vi "host_chunk.vi"() -> ()   [LabVIEW 2020]
doc: "This example demonstrates how to continuously acquire buffered voltage measurements using a DAQmx device.\n\nFor instructions on how to connect your signals to the DAQ device, refer to your device documentation."
uses:
  <vilib>/DAQmx/read.llb/DAQmx Read (Analog Wfm 1Chan NSamp).vi
  <vilib>/DAQmx/create/channels.llb/DAQmx Create Channel (AI-Voltage-Basic).vi
  <vilib>/DAQmx/configure/timing.llb/DAQmx Timing (Sample Clock).vi
  <vilib>/FPGAPlugInAG/cRIO-9040/niLvFpga_Open_cRIO-9040.vi
  <vilib>/rvi/interface/common/dynamic/niFpgaDynamicAddResources.vi
  <vilib>/Utility/error.llb/Error Cluster From Error Code.vi
  <vilib>/rvi/errors/niLvFpgaAdjustHostInterfaceError.vi
  <vilib>/FPGAPlugInAG/Dynamic/niLvFpga_Run_Dynamic.vi
  <vilib>/RVI Host/nirviSupport.llb/nirviErrorClusterFromErrorCode.vi
  <vilib>/DAQmx/miscellaneous.llb/DAQmx Fill In Error Info.vi
  <vilib>/FPGAPlugInAG/Dynamic/niLvFpga_Close_Dynamic.vi
  <vilib>/rvi/interface/nirviOpenFPGA/nirviOpenFPGA.xnode
  FPGA Bitfiles/testDMA_9040_chunk_v1001.lvbitx
  <vilib>/rvi/interface/nirviReadWriteControl/nirviReadWriteControl.xnode
  <vilib>/rvi/interface/nirviMethod/nirviMethod.xnode
  <vilib>/rvi/interface/nirviCloseFPGA/nirviCloseFPGA.xnode
  <resource>/objmgr/daqmx.rc
  <vilib>/rvi/interface/Simulation/niFpgaSimulationCallBeginRW.vi
  <vilib>/rvi/errors/niLvFpgaMergeErrorWithErrorCode.vi
  NiFpgaLv.dll
  <vilib>/FPGAPlugInAG/Dynamic/niLvFpga_WriteFifo_Dynamic.vi
  <vilib>/FPGAPlugInAG/Dynamic/niLvFpga_ReadFifo_Dynamic.vi
  <vilib>/rvi/interface/nirviMethod/StockFPGA_InlinedMethodWaitForSingleIRQ.vi
  <vilib>/FPGAPlugInAG/Dynamic/niLvFpga_WaitOnIrq_Dynamic.vi
  <vilib>/FPGAPlugInAG/Dynamic/niLvFpga_AcknowledgeIrq_Dynamic.vi
panel:
  out "dma read time uS":u32
  out "AvailSampPerChan":u32
  out "write DMA timeout count":i16
  out "uS elapsed":cluster{u32, u32}(graph)
  out "Timed Out":bool
  out "error out":errorcluster
  in  "Stop":bool
  out "Waveform Graph":dbl[][](graph)
  in  "Number of Samples":i32=100
  in  "Sample Rate":dbl=1000.0
  in  "Sample Clock Source":tag="OnboardClock"
  in  "Terminal Configuration":i32(ring)=-1 items=["default"=-1, "RSE"=10083, "NRSE"=10078, "Differential"=10106, "Pseudodifferential"=12529]
  in  "Max Voltage":dbl=5.0
  in  "Min Voltage":dbl=-5.0
  in  "Physical Channel":tag="Mod1/ai0"
  out "Actual Sample Rate":dbl=1000.0 format="%0.2f"
  # "Channel Settings"
  # "Acquired Data"
  # "Timing Settings"
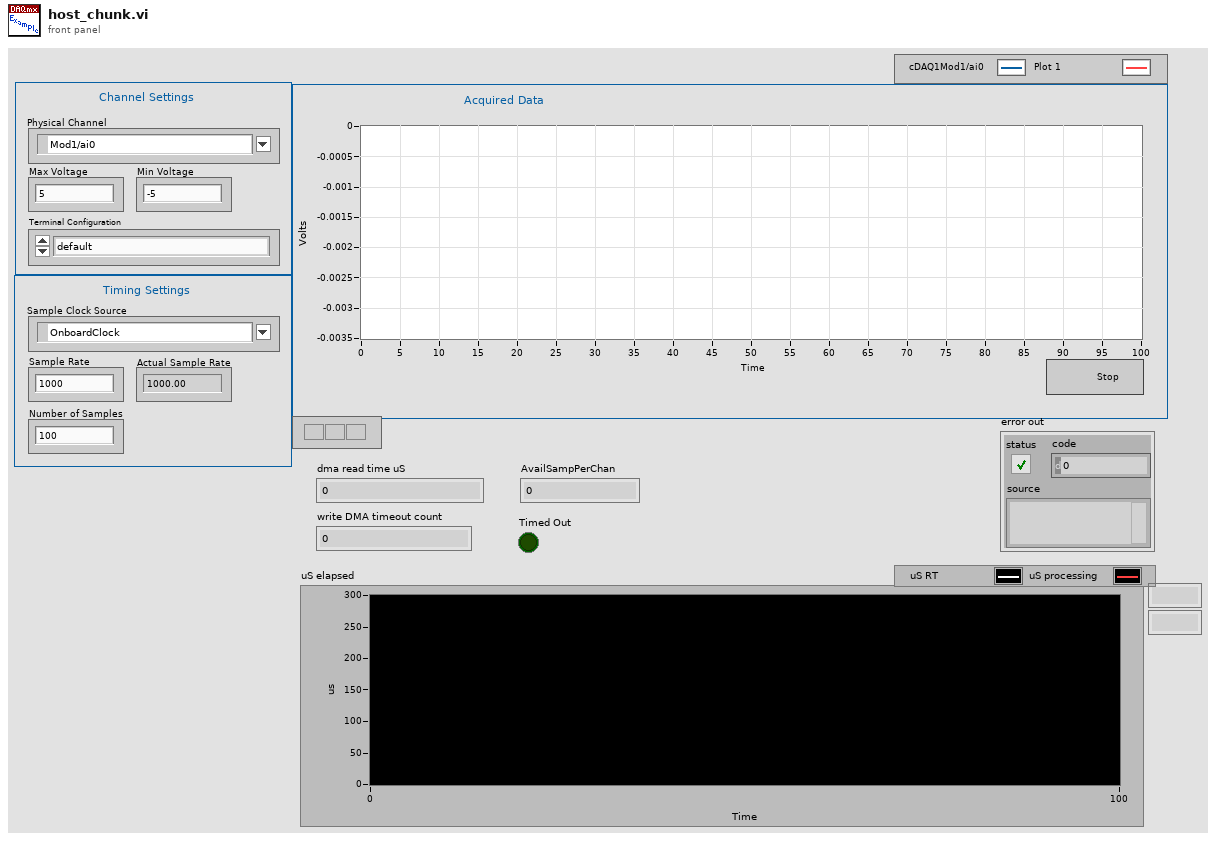
[diagram p1: front panel]
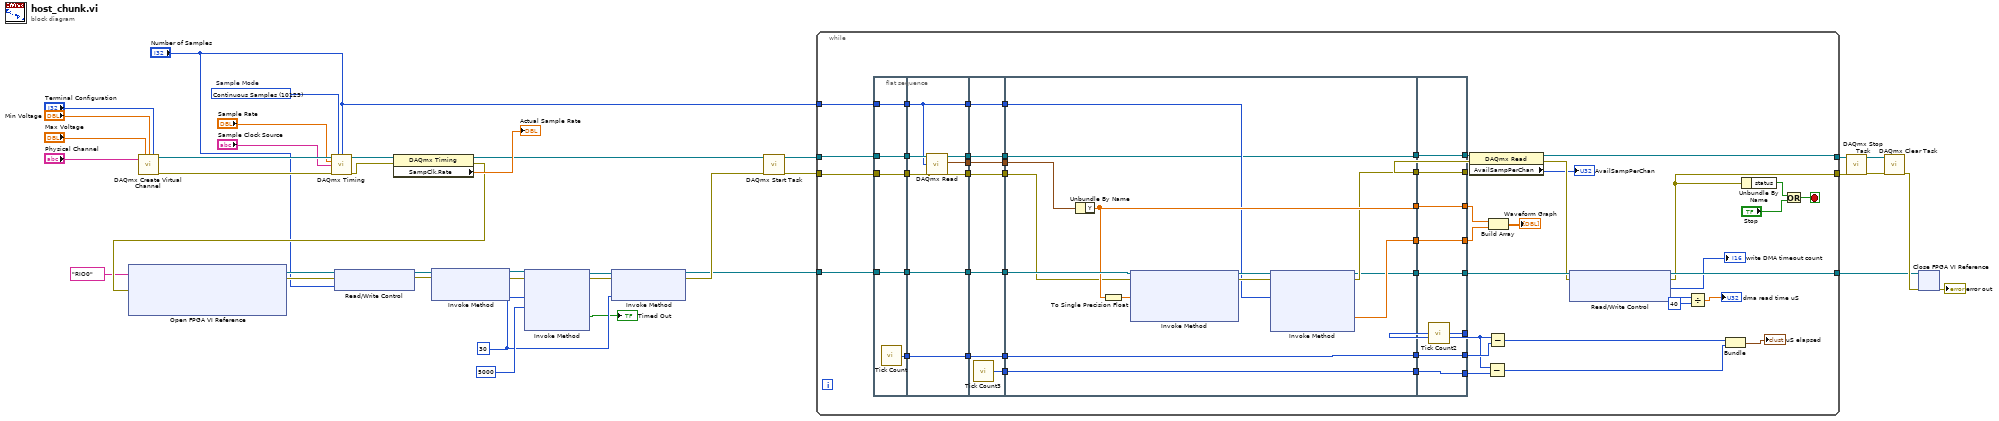
[diagram p0: block diagram]
diagram:
  w5 = u8 30 ("IRQ Number (0)")
  w36 = 10123 items=["Finite Samples"=10178, "Continuous Samples"=10123, "Hardware Timed Single Point"=12522]  # Sample Mode
  n1 = call-poly <vilib>:"DAQmx Create Virtual Channel.vi"("maximum value"="Max Voltage", "minimum value"="Min Voltage", "input terminal configuration"="Terminal Configuration", "physical channels"="Physical Channel") -> ("task out"=w34:refnum<k21>, "error out"=w35:errorcluster)  [unwired: 10 in]
  n2 = call-poly <vilib>:"DAQmx Timing.vi"("task/channels in"=w34, "sample mode"=w36, "samples per channel"="Number of Samples", "rate"="Sample Rate", "source"="Sample Clock Source", "error in"=w35) -> ("task out"=w38:refnum<k21>, "error out"=w37:errorcluster)  [unwired: 8 in]
  n3 = property class="DAQmx Timing"(reference=w38, error in=w37) -> (reference out=w17:refnum<k21>, error out=w18:errorcluster, "SampClk.Rate"=→"Actual Sample Rate":dbl)
  n4 = xnode "Open FPGA VI Reference"("error in"=w18, "resource name"=tag "RIO0") -> ("FPGA VI Reference Out"=w15:refnum<k20>, "error out"=w16:errorcluster)
  n5 = xnode "Read/Write Control"("FPGA VI Reference In"=w15, "error in"=w16, "number of samples"="Number of Samples") -> ("FPGA VI Reference Out"=w12:refnum<k20>, "error out"=w11:errorcluster)
  n6 = xnode "Invoke Method"("FPGA VI Reference In"=w12, "error in"=w11) -> ("FPGA VI Reference Out"=w10:refnum<k20>, "error out"=w9:errorcluster)  [unwired: 1 in]
  n7 = xnode "Invoke Method"("FPGA VI Reference In"=w10, "error in"=w9, "IRQ Number(s)"=w5, "Timeout (ms)"=5000) -> ("FPGA VI Reference Out"=w8:refnum<k20>, "error out"=w7:errorcluster, "Timed Out"=→"Timed Out":bool)  [unwired: 1 out]
  n8 = xnode "Invoke Method"("FPGA VI Reference In"=w8, "error in"=w7, "IRQ Number(s)"=w5) -> ("FPGA VI Reference Out"=w2:refnum<k20>, "error out"=w3:errorcluster)
  n9 = call <vilib>:"DAQmx Start Task.vi"("task/channels in"=w17, "error in"=w3) -> ("task out"=w33:refnum<k21>, "error out"=w32:errorcluster)  [unwired: 12 in]
  n10 = while {
    tunnel: w33 -> [w91]
    tunnel: w32 -> [w86]
    tunnel: [w68] -> w24
    tunnel: [w71] -> w23
    tunnel: "Number of Samples" -> [w56]
    tunnel: w2 -> [w85]
    tunnel: [w72] -> w1
    stop <- w87 stop-if-true
    n11 = flat-sequence {
      tunnel: w91 -> [w96]
      tunnel: [w96] -> w61
      tunnel: [w95] -> w60
      tunnel: w86 -> [w95]
      tunnel: [w94] -> w59
      tunnel: w85 -> [w94]
      tunnel: [w93] -> w58
      tunnel: [w92] -> w57
      tunnel: w56 -> [w92]
      tunnel: w61 -> [w102]
      tunnel: [w102] -> w55
      tunnel: w60 -> [w101]
      tunnel: [w101] -> w53
      tunnel: w59 -> [w100]
      tunnel: [w100] -> w51
      tunnel: w58 -> [w99]
      tunnel: [w99] -> w49
      tunnel: [w98] -> w47
      tunnel: w57 -> [w97]
      tunnel: [w97] -> w45
      tunnel: w55 -> [w109]
      tunnel: [w109] -> w54
      tunnel: w53 -> [w108]
      tunnel: [w108] -> w52
      tunnel: w51 -> [w107]
      tunnel: [w107] -> w50
      tunnel: w49 -> [w106]
      tunnel: [w106] -> w48
      tunnel: w47 -> [w105]
      tunnel: [w105] -> w46
      tunnel: w45 -> [w104]
      tunnel: [w104] -> w44
      tunnel: [w103] -> w40
      tunnel: w54 -> [w111]
      tunnel: w52 -> [w112]
      tunnel: w50 -> [w123]
      tunnel: [w111] -> w80
      tunnel: [w117] -> w79
      tunnel: [w119] -> w78
      tunnel: [w118] -> w77
      tunnel: [w116] -> w76
      tunnel: [w115] -> w74
      tunnel: w48 -> [w115]
      tunnel: w46 -> [w114]
      tunnel: w44 -> [w113]
      tunnel: [w110] -> w41
      tunnel: w40 -> [w110]
      tunnel: [w127] -> w81
      tunnel: [w128] -> w84
      tunnel: [w129] -> w83
      tunnel: [w130] -> w67
      tunnel: [w131] -> w90
      tunnel: w80 -> [w131]
      tunnel: w79 -> [w130]
      tunnel: w78 -> [w129]
      tunnel: w77 -> [w128]
      tunnel: w76 -> [w127]
      tunnel: [w126] -> w43
      tunnel: [w125] -> w75
      tunnel: w74 -> [w125]
      tunnel: [w124] -> w42
      tunnel: w41 -> [w124]
      frame #0 {
        n12 = call "Tick Count"() -> ("Tick Count(uSec)"=w93:u32)
      }
      frame #1 {
        n13 = call-poly <vilib>:"DAQmx Read.vi"("task/channels in"=w102, "number of samples per channel"=w97, "error in"=w101) -> ("data"=w98:waveform(dbl))  [unwired: 10 in, 2 out]
      }
      frame #2 {
        n14 = call "Tick Count3"() -> ("Tick Count(uSec)"=w103:u32)
      }
      frame #3 {
        n15 = Unbundle By Name(w114) -> ("Y"=w118:dbl[])
        n16 = To Single Precision Float(number=w118) -> (single precision float=w122:sgl[])
        n17 = xnode "Invoke Method"("FPGA VI Reference In"=w123, "error in"=w112, "Data"=w122) -> ("FPGA VI Reference Out"=w121:refnum<k20>, "error out"=w120:errorcluster)  [unwired: 1 in, 1 out]
        n18 = xnode "Invoke Method"("FPGA VI Reference In"=w121, "error in"=w120, "Number of Elements"=w113) -> ("FPGA VI Reference Out"=w116:refnum<k20>, "error out"=w117:errorcluster, "Data"=w119:sgl[])  [unwired: 1 in, 1 out]
      }
      frame #4 {
        n19 = call "Tick Count2"() -> ("Tick Count(uSec)"=w126:u32)
      }
    }
    n20 = property class="DAQmx Read"(reference=w90, error in=w67) -> (reference out=w68:refnum<k21>, error out=w66:errorcluster, "AvailSampPerChan"=→"AvailSampPerChan":u32)
    n21 = Subtract(x=w43, y=w42) -> (x-y=w39:u32)
    n22 = Subtract(x=w43, y=w75) -> (x-y=w73:u32)
    n23 = Build Array(w84, w83) -> (→"Waveform Graph":dbl[][])
    n24 = xnode "Read/Write Control"("FPGA VI Reference In"=w81, "error in"=w66) -> ("FPGA VI Reference Out"=w72:refnum<k20>, "error out"=w71:errorcluster, "write DMA timeout count"=→"write DMA timeout count":i16, "dma read time ticks"=w64:u32)
    n25 = Divide(x=w64, y=u32 40) -> (x/y=→"dma read time uS":dbl)
    n26 = Bundle(w73, w39) -> (→"uS elapsed":cluster{u32, u32})  [unwired: 1 in]
    n27 = Unbundle By Name(w71) -> ("status"=w88:bool)
    n28 = Or(x=w88, y="Stop") -> (x .or. y?=w87:bool)
  }
  n29 = call <vilib>:"DAQmx Stop Task.vi"("task/channels in"=w24, "error in"=w23) -> ("task out"=w21:refnum<k21>, "error out"=w22:errorcluster)  [unwired: 12 in]
  n30 = call <vilib>:"DAQmx Clear Task.vi"("task in"=w21, "error in"=w22) -> ("error out"=w20:errorcluster)  [unwired: 13 in]
  n31 = xnode "Close FPGA VI Reference"("FPGA VI Reference In"=w1, "error in"=w20) -> ("error out"=→"error out":errorcluster)
